vi "ScanDelayGetMinMaxCurrTriggerIn.vi"(8 "error in (no error)":errorcluster, 9 "wait":u32=10, 11 "VISA resource name in":refnum<visa-resource-name>) -> (0 "error out":errorcluster, 2 "value":i32, 3 "VISA resource name out":refnum<visa-resource-name>, 4 "min":i32, 5 "max":i32)   [LabVIEW 2018]
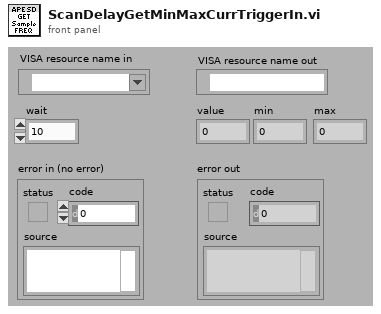
[diagram p1: front panel]
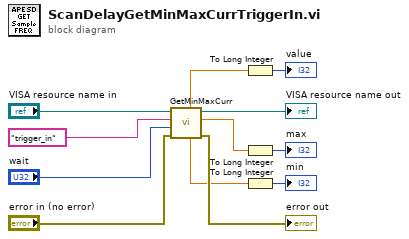
[diagram p0: block diagram]
diagram:
  n1 = call "GetMinMaxCurr.vi"("VISA resource name in"="VISA resource name in", "parameter"="trigger_in", "wait"="wait", "error in (no error)"="error in (no error)") -> ("value"=w5:dbl, "MIN"=w4:dbl, "VISA resource name out"=→"VISA resource name out":refnum<visa-resource-name>, "MAX"=w6:dbl, "error out"=→"error out":errorcluster)  [unwired: 2 in]
  n2 = To Long Integer(number=w5) -> (32bit integer=→"value":i32)
  n3 = To Long Integer(number=w6) -> (32bit integer=→"max":i32)
  n4 = To Long Integer(number=w4) -> (32bit integer=→"min":i32)
